vi "Gear Strip Detection.vi"(0 "Red or Hue Range (Detect Green)":cluster{"Lower value":i32, "Upper value":i32}={"Lower value"=100, "Upper value"=160}, 1 "Green or Sat Range (Detect Green)":cluster{"Lower value":i32, "Upper value":i32}={"Lower value"=0, "Upper value"=255}, 2 "Blue or Luma or Val or Inten Range (Detect Green)":cluster{"Lower value":i32, "Upper value":i32}={"Lower value"=205, "Upper value"=255}, 7 "error in":errorcluster) -> (20 "Number of Matches (Strip Detection)":i32, 21 "Shape Report (Strip Detection)":T2(array[cluster]) {"Score" format="%.2f"; "Centroid"."y" format="%.2f"; "Centroid"."x" format="%.2f"}, 22 "Shape Report (calibrated) (Strip Detection)":T2(array[cluster]) {"Score" format="%.2f"; "Centroid"."y" format="%.2f"; "Centroid"."x" format="%.2f"}, 27 "error out":errorcluster)   [LabVIEW 2016]
uses:
  <vilib>/vision/driver/NI_Vision_Acquisition_Software.lvlib
  <vilib>/vision/NI_Vision_Development_Module.lvlib
panel:
  out "Image Out":T1(plugin-control)
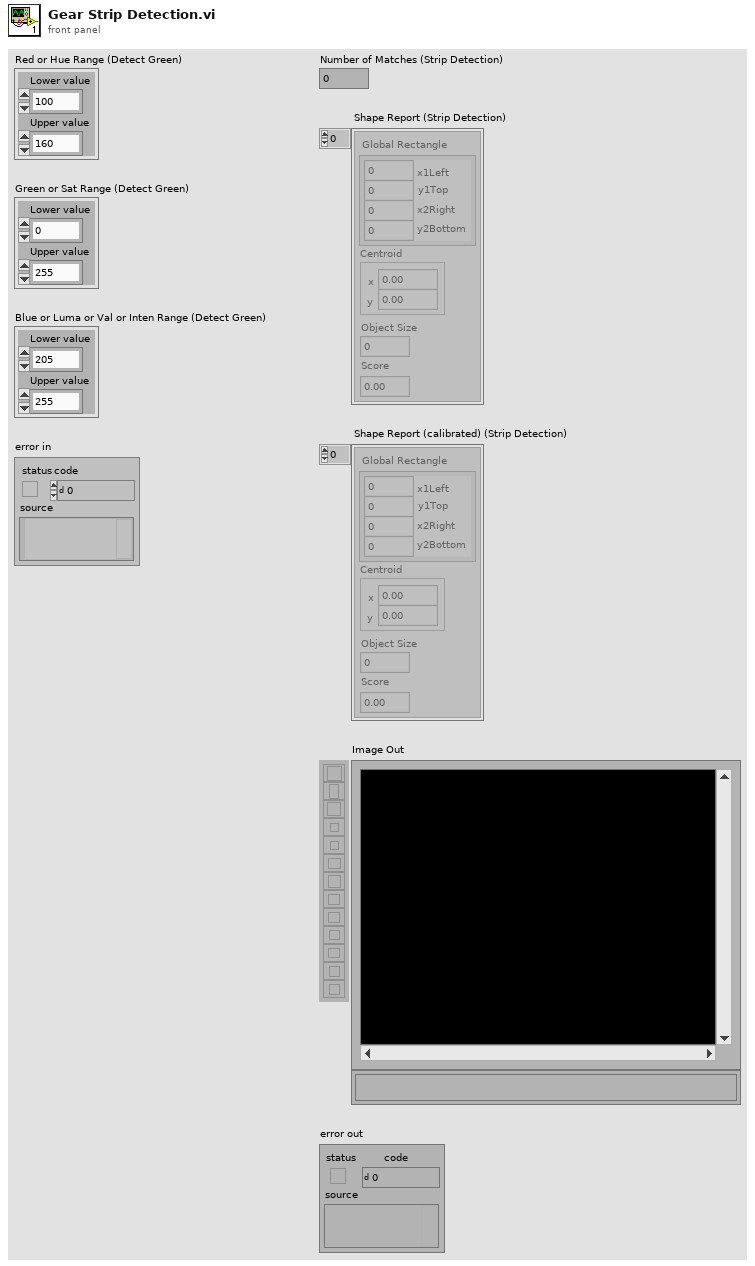
[diagram p1: front panel]
types:
  T1 = typedef "IMAQ Image.ctl" = refnum<image>
  T2 = cluster{"Global Rectangle":cluster{"x1Left":i32, "y1Top":i32, "x2Right":i32, "y2Bottom":i32}, "Centroid":cluster{"x":sgl, "y":sgl}, "Object Size":u32, "Score":dbl}[]
  T3 = cluster{"Measurement Parameter":i32, "Range Lower Value":dbl, "Range Upper Value":dbl, "Range":bool, "Measurement Type":bool}[]
  T4 = typedef "IMAQdx.ctl" = refnum<k21>
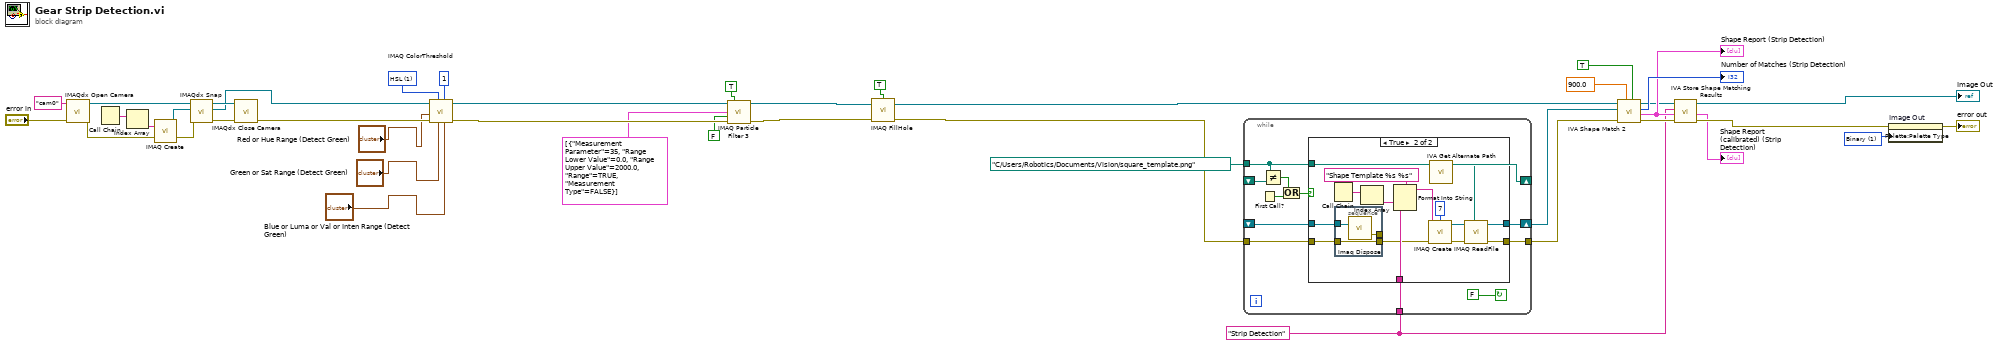
[diagram p0: block diagram]
diagram:
  w1 = u32 1 items=["Grayscale", "Binary", "Gradient", "Rainbow", "Temperature", "User Defined", "Binary 16 Bit", "Gradient 16 Bit", "Rainbow 16 Bit", "Temperature 16 Bit", "User Defined 16 Bit"] ("Palette Type")
  w4 = "Strip Detection" ("Step Name")
  w30 = u16 1 items=["RGB", "HSL", "HSV", "HSI"] ("Color Mode")
  n1 = call <vilib>:"IMAQdx Open Camera.vi"("error in"="error in", "Session In"="cam0" ("Interface Name")) -> ("error out"=w41:errorcluster, "Session Out"=w35:T4)  [unwired: 1 in, 7 out]
  n2 = Call Chain() -> (call chain=w33:string[])
  n3 = Index Array(array=w33) -> (element=w32:string)  [unwired: 1 in]
  n4 = call "IMAQ Create"("Image Name"=w32, "error in (no error)"=w41) -> ("New Image"=w37:T1, "error out"=w36:errorcluster)  [unwired: 2 in, 1 out]
  n5 = call <vilib>:"IMAQdx Snap.vi"("error in"=w36, "Image In"=w37, "Session In"=w35) -> ("error out"=w39:errorcluster, "Image Out"=w26:T1, "Session Out"=w40:T4)  [unwired: 6 out]
  n6 = call <vilib>:"IMAQdx Close Camera.vi"("error in"=w39, "Session In"=w40) -> ("error out"=w38:errorcluster)  [unwired: 9 out]
  n7 = call "IMAQ ColorThreshold"("Blue or Luma or Val or Inten Range"="Blue or Luma or Val or Inten Range (Detect Green)", "Replace Value"=1, "Green or Sat Range"="Green or Sat Range (Detect Green)", "Color Mode"=w30, "error in (no error)"=w38, "Red or Hue Range"="Red or Hue Range (Detect Green)", "Image Src"=w26) -> ("error out"=w25:errorcluster, "Image Dst Out"=w21:T1)  [unwired: 1 in, 2 out]
  n8 = call "IMAQ Particle Filter 3"("Image Src"=w21, "Connectivity 4/8 (8)"=TRUE, "Selection Values"=T3 [{"Measurement Parameter"=35, "Range Lower Value"=0.0, "Range Upper Value"=2000.0, "Range"=TRUE, "Measurement Type"=FALSE}], "Keep/Remove Particles (F)"=FALSE ("Keep/Remove Particles"), "error in (no error)"=w25) -> ("Image Dst Out"=w18:T1, "error out"=w22:errorcluster)  [unwired: 4 in, 5 out]
  n9 = call "IMAQ FillHole"("error in (no error)"=w22, "Image Src"=w18, "Connectivity 4/8 (8)"=TRUE) -> ("error out"=w17:errorcluster, "Image Dst Out"=w13:T1)  [unwired: 1 in, 2 out]
  n10 = while {
    shift-right: [w53] -> w5
    shift-left: _ -> [w52]
    tunnel: [w50] -> w6
    tunnel: w17 -> [w49]
    tunnel: path "C:/Users/Robotics/Documents/Vision/square_template.png" ("Template Path") -> [w47]
    tunnel: w4 -> [w48]
    shift-right: [w47] -> _
    shift-left: _ -> [w46]
    stop <- FALSE continue-if-true
    n11 = First Call?() -> (First Call?: T/F=w45:bool)
    n12 = Not Equal?(x=w47, y=w46) -> (x != y?=w44:bool)
    n13 = Or(x=w44, y=w45) -> (x .or. y?=w43:bool)
    n14 = case shown="True" w43 {
      tunnel: [w55 w67] -> w53
      tunnel: w52 -> [w55 w58]
      tunnel: [w54 w65] -> w50
      tunnel: w49 -> [w54 w57]
      tunnel: w47 -> [_ w60]
      tunnel: w48 -> [_ w61]
      frame False {
      }
      frame True {
        n15 = Call Chain() -> (call chain=w63:string[])
        n16 = stacked-sequence {
          tunnel: w58 -> [w73]
          tunnel: w57 -> [w72]
          tunnel: [w72] -> w56
          tunnel: [w71] -> _
          frame #0 {
            n17 = call "Imaq Dispose"("Image"=w73) -> ("error out"=w71:errorcluster)  [unwired: 2 in, 3 out]
          }
        }
        n18 = Index Array(array=w63) -> (element=w62:string)  [unwired: 1 in]
        n19 = Format Into String(format string="Shape Template %s %s" ("Image Name"), w62, w61) -> (resulting string=w70:string)  [unwired: 2 in, 1 out]
        n20 = call "IMAQ Create"("Border Size"=7, "Image Name"=w70, "error in (no error)"=w56) -> ("New Image"=w68:T1, "error out"=w66:errorcluster)  [unwired: 1 in, 1 out]
        n21 = call <vilib>:"IVA Get Alternate Path.vi"("Path In"=w60) -> ("Path Out"=w59:path)  [unwired: 10 out]
        n22 = call "IMAQ ReadFile"("File Path"=w59, "error in (no error)"=w66, "Image"=w68) -> ("error out"=w65:errorcluster, "Image Out"=w67:T1)  [unwired: 2 in, 5 out]
      }
    }
  }
  n23 = call <vilib>:"IVA Shape Match 2.vi"("Scale Invariance"=TRUE, "Minimal Score"=900.0, "error in (no error)"=w6, "Template"=w5, "Image Src"=w13) -> ("error out"=w12:errorcluster, "Shape Report"=w10:T2, "Number of Matches"=→"Number of Matches (Strip Detection)":i32, "Image Out"=w9:T1)  [unwired: 3 out]
  "Shape Report (Strip Detection)" <- w10
  n24 = call <vilib>:"IVA Store Shape Matching Results.vi"("error in (no error)"=w12, "Shape Report"=w10, "Step Name"=w4, "Image in"=w9) -> ("error out"=w11:errorcluster, "Shape Report (calibrated)"=→"Shape Report (calibrated) (Strip Detection)":T2, "Image dup"=→"Image Out":T1)  [unwired: 5 out]
  n25 = property on="Image Out" class="ImageControl"(error in=w11, "Palette:Palette Type"=w1) -> (error out=→"error out":errorcluster)  [unwired: 1 in, 1 out]
